vi "Add to Tree (Internal).vi"(6 "Display Text Override":string, 7 "Add children? (F)":bool, 8 "error in (no error)":errorcluster, 9 "Parent Tag":string, 10 "Tree Manager in":refnum<class "Tree Manager.lvclass">, 11 "Data Item in":refnum<class "Data Item.lvclass">) -> (0 "error out":errorcluster, 1 "New Tag":string, 2 "Tree Manager out":refnum<class "Tree Manager.lvclass">, 3 "Data Item out":refnum<class "Data Item.lvclass">)   [LabVIEW 2020, in "VILab.lvlib" / "Data Item.lvclass"]
uses:
  Data Item.lvclass
  Tree Manager/Tree Manager.lvclass
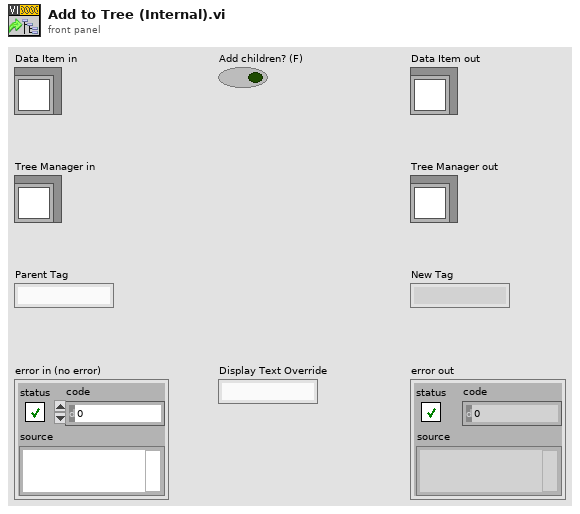
[diagram p1: front panel]
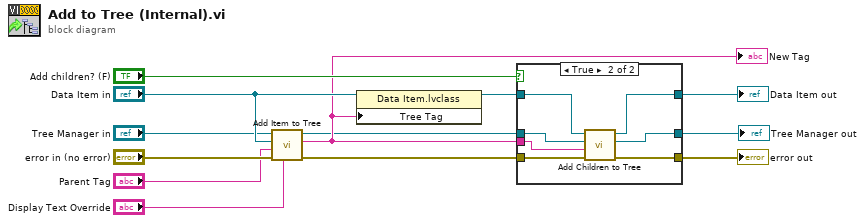
[diagram p0: block diagram]
diagram:
  n1 = call "Add Item to Tree.vi"("Display Text Override"="Display Text Override", "error in (no error)"="error in (no error)", "Parent Tag"="Parent Tag", "Data Item"="Data Item in", "Tree Manager in"="Tree Manager in") -> ("error out"=w2:errorcluster, "New Tag"=w4:string, "Tree Manager out"=w3:refnum<class "Tree Manager.lvclass">)  [unwired: 4 in]
  "New Tag" <- w4
  n2 = property class="Data Item.lvclass"(reference="Data Item in", "Tree Tag"=w4) -> (reference out=w1:refnum<class "Data Item.lvclass">)  [unwired: 1 in, 1 out]
  n3 = case shown="True" "Add children? (F)" {
    tunnel: w3 -> [w15 w23]
    tunnel: w2 -> [w14 w21]
    tunnel: w4 -> [_ w22]
    tunnel: [w15 w19] -> w7
    tunnel: w1 -> [w16 w17]
    tunnel: [w16 w20] -> w10
    tunnel: [w14 w18] -> w12
    frame False {
    }
    frame True {
      n4 = call "Add Children to Tree.vi"("error in (no error)"=w21, "Parent Tag"=w22, "Tree Manager in"=w23, "Data Item in"=w17) -> ("error out"=w18:errorcluster, "Tree Manager out"=w19:refnum<class "Tree Manager.lvclass">, "Data Item out"=w20:refnum<class "Data Item.lvclass">)  [unwired: 5 in]
    }
  }
  "error out" <- w12
  "Data Item out" <- w10
  "Tree Manager out" <- w7
